vi "Reader Encoder.vi"() -> ()   [LabVIEW 2011]
uses:
  <vilib>/Utility/file.llb/Read From Spreadsheet File (DBL).vi
panel:
  out "Slide 2":dbl(slide) scale=-1000.0..1000.0
  out "Slide":dbl(slide) scale=-1000.0..1000.0
  in  "File":bool
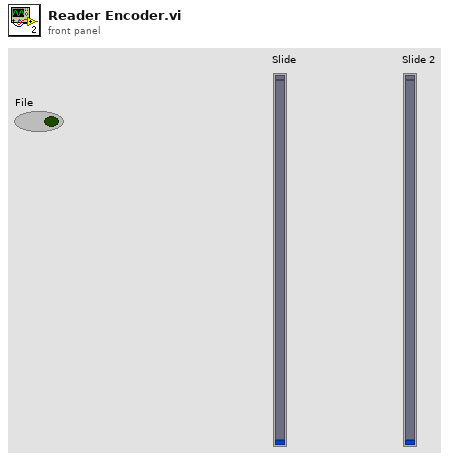
[diagram p1: front panel]
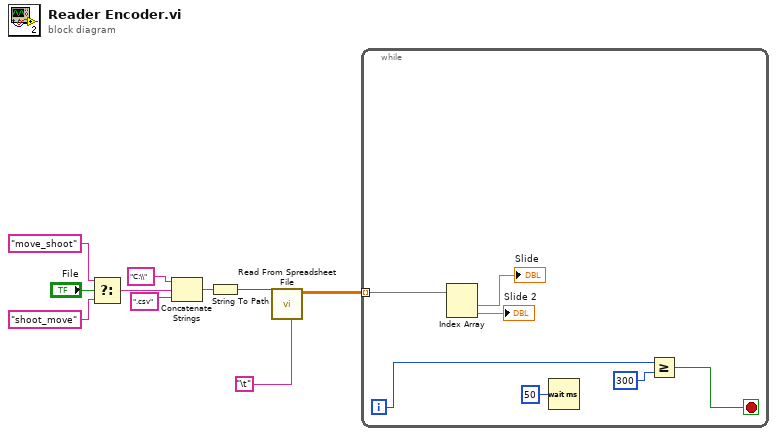
[diagram p0: block diagram]
diagram:
  n1 = Select(t="move_shoot", s="File", f="shoot_move") -> (s? t:f=w5:string)
  n2 = Concatenate Strings("C:\\", w5, ".csv") -> (w4:string)
  n3 = String To Path(string=w4) -> (path=w3:path)
  n4 = call-poly <vilib>:"Read From Spreadsheet File.vi"("delimiter (\\t)"="\t", "file path (dialog if empty)"=w3) -> ("all rows"=w1:dbl[][])  [unwired: 5 in, 4 out]
  n5 = while {
    tunnel: w1 -> [w13] mode=indexing
    i -> [w16]
    stop <- w14 stop-if-true
    n6 = Index Array(array=w13) -> (element #1=→"Slide":dbl, element #2=→"Slide 2":dbl)  [unwired: 2 in]
    n7 = Wait (ms)(milliseconds to wait=u32 50) -> ()  [unwired: 1 out]
    n8 = Greater Or Equal?(x=w16, y=300) -> (x >= y?=w14:bool)
  }
